vi "メイン.vi"() -> (2 "測定周期/ms":dbl, 3 "値転記用配列":T2[](array[typedef]))   [LabVIEW 2021] (continued)
                      n6047 = property on="MAX/MINグローバルリセット用" class="Arr (指定)"() -> ("Value"=w8245:string[][])  [unwired: 2 in, 2 out]
                      n6048 = global write "測定値MAXMIN_G.vi" "測定値MAX/MINグローバル"(w8245) -> ()
                    }
                  }
                  n6049 = case shown="FALSE" w8244 {
                    frame False {
                    }
                    frame True {
                      n6050 = property on="MAX/MINグローバルリセット用" class="Arr (指定)"() -> ("Value"=w8246:string[][])  [unwired: 2 in, 2 out]
                      n6051 = global write "測定値MAXMIN_G.vi" "測定値MAX/MINグローバル"(w8246) -> ()
                    }
                  }
                }
                frame 1 {
                  n6052 = local read "測定新値\nリセット用 2"() -> (w8247:bool)
                  n6053 = local read "測定旧値 2"() -> (w8248:bool)
                  n6054 = case shown="FALSE" w8247 {
                    frame False {
                    }
                    frame True {
                      n6055 = property on="MAX/MINグローバルリセット用" class="Arr (指定)"() -> ("Value"=w8249:string[][])  [unwired: 2 in, 2 out]
                      n6056 = global write "測定値MAXMIN_G.vi" "測定値MAX/MINグローバル"(w8249) -> ()
                    }
                  }
                  n6057 = case shown="FALSE" w8248 {
                    frame False {
                    }
                    frame True {
                      n6058 = property on="MAX/MINグローバルリセット用" class="Arr (指定)"() -> ("Value"=w8250:string[][])  [unwired: 2 in, 2 out]
                      n6059 = global write "測定値MAXMIN_G.vi" "測定値MAX/MINグローバル"(w8250) -> ()
                    }
                  }
                }
                frame 2 {
                  n6060 = local read "測定新値\nリセット用 3"() -> (w8251:bool)
                  n6061 = local read "測定旧値 3"() -> (w8252:bool)
                  n6062 = case shown="FALSE" w8251 {
                    frame False {
                    }
                    frame True {
                      n6063 = property on="MAX/MINグローバルリセット用" class="Arr (指定)"() -> ("Value"=w8253:string[][])  [unwired: 2 in, 2 out]
                      n6064 = global write "測定値MAXMIN_G.vi" "測定値MAX/MINグローバル"(w8253) -> ()
                    }
                  }
                  n6065 = case shown="FALSE" w8252 {
                    frame False {
                    }
                    frame True {
                      n6066 = property on="MAX/MINグローバルリセット用" class="Arr (指定)"() -> ("Value"=w8254:string[][])  [unwired: 2 in, 2 out]
                      n6067 = global write "測定値MAXMIN_G.vi" "測定値MAX/MINグローバル"(w8254) -> ()
                    }
                  }
                }
                frame 3 {
                  n6068 = local read "測定新値\nリセット用 4"() -> (w8255:bool)
                  n6069 = local read "測定旧値 4"() -> (w8256:bool)
                  n6070 = case shown="FALSE" w8255 {
                    frame False {
                    }
                    frame True {
                      n6071 = property on="MAX/MINグローバルリセット用" class="Arr (指定)"() -> ("Value"=w8257:string[][])  [unwired: 2 in, 2 out]
                      n6072 = global write "測定値MAXMIN_G.vi" "測定値MAX/MINグローバル"(w8257) -> ()
                    }
                  }
                  n6073 = case shown="FALSE" w8256 {
                    frame False {
                    }
                    frame True {
                      n6074 = property on="MAX/MINグローバルリセット用" class="Arr (指定)"() -> ("Value"=w8258:string[][])  [unwired: 2 in, 2 out]
                      n6075 = global write "測定値MAXMIN_G.vi" "測定値MAX/MINグローバル"(w8258) -> ()
                    }
                  }
                }
                frame 4 {
                  n6076 = local read "測定新値\nリセット用 5"() -> (w8259:bool)
                  n6077 = local read "測定旧値 5"() -> (w8260:bool)
                  n6078 = case shown="FALSE" w8259 {
                    frame False {
                    }
                    frame True {
                      n6079 = property on="MAX/MINグローバルリセット用" class="Arr (指定)"() -> ("Value"=w8261:string[][])  [unwired: 2 in, 2 out]
                      n6080 = global write "測定値MAXMIN_G.vi" "測定値MAX/MINグローバル"(w8261) -> ()
                    }
                  }
                  n6081 = case shown="FALSE" w8260 {
                    frame False {
                    }
                    frame True {
                      n6082 = property on="MAX/MINグローバルリセット用" class="Arr (指定)"() -> ("Value"=w8262:string[][])  [unwired: 2 in, 2 out]
                      n6083 = global write "測定値MAXMIN_G.vi" "測定値MAX/MINグローバル"(w8262) -> ()
                    }
                  }
                }
                frame 5 {
                  n6084 = local read "測定新値\nリセット用 6"() -> (w8263:bool)
                  n6085 = local read "測定旧値 6"() -> (w8264:bool)
                  n6086 = case shown="FALSE" w8263 {
                    frame False {
                    }
                    frame True {
                      n6087 = property on="MAX/MINグローバルリセット用" class="Arr (指定)"() -> ("Value"=w8265:string[][])  [unwired: 2 in, 2 out]
                      n6088 = global write "測定値MAXMIN_G.vi" "測定値MAX/MINグローバル"(w8265) -> ()
                    }
                  }
                  n6089 = case shown="FALSE" w8264 {
                    frame False {
                    }
                    frame True {
                      n6090 = property on="MAX/MINグローバルリセット用" class="Arr (指定)"() -> ("Value"=w8266:string[][])  [unwired: 2 in, 2 out]
                      n6091 = global write "測定値MAXMIN_G.vi" "測定値MAX/MINグローバル"(w8266) -> ()
                    }
                  }
                }
                frame 6 {
                  n6092 = local read "測定新値\nリセット用 7"() -> (w8267:bool)
                  n6093 = local read "測定旧値 7"() -> (w8268:bool)
                  n6094 = case shown="FALSE" w8267 {
                    frame False {
                    }
                    frame True {
                      n6095 = property on="MAX/MINグローバルリセット用" class="Arr (指定)"() -> ("Value"=w8269:string[][])  [unwired: 2 in, 2 out]
                      n6096 = global write "測定値MAXMIN_G.vi" "測定値MAX/MINグローバル"(w8269) -> ()
                    }
                  }
                  n6097 = case shown="FALSE" w8268 {
                    frame False {
                    }
                    frame True {
                      n6098 = property on="MAX/MINグローバルリセット用" class="Arr (指定)"() -> ("Value"=w8270:string[][])  [unwired: 2 in, 2 out]
                      n6099 = global write "測定値MAXMIN_G.vi" "測定値MAX/MINグローバル"(w8270) -> ()
                    }
                  }
                }
                frame 7 {
                  n6100 = local read "測定新値\nリセット用 8"() -> (w8271:bool)
                  n6101 = local read "測定旧値 8"() -> (w8272:bool)
                  n6102 = case shown="FALSE" w8271 {
                    frame False {
                    }
                    frame True {
                      n6103 = property on="MAX/MINグローバルリセット用" class="Arr (指定)"() -> ("Value"=w8273:string[][])  [unwired: 2 in, 2 out]
                      n6104 = global write "測定値MAXMIN_G.vi" "測定値MAX/MINグローバル"(w8273) -> ()
                    }
                  }
                  n6105 = case shown="FALSE" w8272 {
                    frame False {
                    }
                    frame True {
                      n6106 = property on="MAX/MINグローバルリセット用" class="Arr (指定)"() -> ("Value"=w8274:string[][])  [unwired: 2 in, 2 out]
                      n6107 = global write "測定値MAXMIN_G.vi" "測定値MAX/MINグローバル"(w8274) -> ()
                    }
                  }
                }
                frame 8 {
                  n6108 = local read "測定新値\nリセット用 9"() -> (w8275:bool)
                  n6109 = local read "測定旧値 9"() -> (w8276:bool)
                  n6110 = case shown="FALSE" w8275 {
                    frame False {
                    }
                    frame True {
                      n6111 = property on="MAX/MINグローバルリセット用" class="Arr (指定)"() -> ("Value"=w8277:string[][])  [unwired: 2 in, 2 out]
                      n6112 = global write "測定値MAXMIN_G.vi" "測定値MAX/MINグローバル"(w8277) -> ()
                    }
                  }
                  n6113 = case shown="FALSE" w8276 {
                    frame False {
                    }
                    frame True {
                      n6114 = property on="MAX/MINグローバルリセット用" class="Arr (指定)"() -> ("Value"=w8278:string[][])  [unwired: 2 in, 2 out]
                      n6115 = global write "測定値MAXMIN_G.vi" "測定値MAX/MINグローバル"(w8278) -> ()
                    }
                  }
                }
                frame 10 {
                  n6116 = local read "測定新値\nリセット用 11"() -> (w8279:bool)
                  n6117 = local read "測定旧値 11"() -> (w8280:bool)
                  n6118 = case shown="FALSE" w8279 {
                    frame False {
                    }
                    frame True {
                      n6119 = property on="MAX/MINグローバルリセット用" class="Arr (指定)"() -> ("Value"=w8281:string[][])  [unwired: 2 in, 2 out]
                      n6120 = global write "測定値MAXMIN_G.vi" "測定値MAX/MINグローバル"(w8281) -> ()
                    }
                  }
                  n6121 = case shown="FALSE" w8280 {
                    frame False {
                    }
                    frame True {
                      n6122 = property on="MAX/MINグローバルリセット用" class="Arr (指定)"() -> ("Value"=w8282:string[][])  [unwired: 2 in, 2 out]
                      n6123 = global write "測定値MAXMIN_G.vi" "測定値MAX/MINグローバル"(w8282) -> ()
                    }
                  }
                }
                frame 11 {
                  n6124 = local read "測定新値\nリセット用 12"() -> (w8283:bool)
                  n6125 = local read "測定旧値 12"() -> (w8284:bool)
                  n6126 = case shown="FALSE" w8283 {
                    frame False {
                    }
                    frame True {
                      n6127 = property on="MAX/MINグローバルリセット用" class="Arr (指定)"() -> ("Value"=w8285:string[][])  [unwired: 2 in, 2 out]
                      n6128 = global write "測定値MAXMIN_G.vi" "測定値MAX/MINグローバル"(w8285) -> ()
                    }
                  }
                  n6129 = case shown="FALSE" w8284 {
                    frame False {
                    }
                    frame True {
                      n6130 = property on="MAX/MINグローバルリセット用" class="Arr (指定)"() -> ("Value"=w8286:string[][])  [unwired: 2 in, 2 out]
                      n6131 = global write "測定値MAXMIN_G.vi" "測定値MAX/MINグローバル"(w8286) -> ()
                    }
                  }
                }
              }
            }
          }
          frame #1 {
            w8287 = FALSE
            # "②測定新規リセット用、測定旧値のリセット"
            n6132 = for {
              N: w8288 -> [_]
              tunnel: w8287 -> [w8292]
              i -> [w8293]
              n6133 = case shown="11" w8293 {
                tunnel: w8292 -> [w8294 w8295 w8296 w8297 w8298 w8299 w8300 w8301 w8302 w8303 w8304 w8305]
                frame 0, Default {
                  n6134 = local write "測定新値\nリセット用 1"(w8294) -> ()
                  n6135 = local write "測定旧値 1"(w8294) -> ()
                }
                frame 1 {
                  n6136 = local write "測定新値\nリセット用 2"(w8295) -> ()
                  n6137 = local write "測定旧値 2"(w8295) -> ()
                }
                frame 2 {
                  n6138 = local write "測定新値\nリセット用 3"(w8296) -> ()
                  n6139 = local write "測定旧値 3"(w8296) -> ()
                }
                frame 3 {
                  n6140 = local write "測定新値\nリセット用 4"(w8297) -> ()
                  n6141 = local write "測定旧値 4"(w8297) -> ()
                }
                frame 4 {
                  n6142 = local write "測定新値\nリセット用 5"(w8298) -> ()
                  n6143 = local write "測定旧値 5"(w8298) -> ()
                }
                frame 5 {
                  n6144 = local write "測定新値\nリセット用 6"(w8299) -> ()
                  n6145 = local write "測定旧値 6"(w8299) -> ()
                }
                frame 6 {
                  n6146 = local write "測定新値\nリセット用 7"(w8300) -> ()
                  n6147 = local write "測定旧値 7"(w8300) -> ()
                }
                frame 7 {
                  n6148 = local write "測定新値\nリセット用 8"(w8301) -> ()
                  n6149 = local write "測定旧値 8"(w8301) -> ()
                }
                frame 8 {
                  n6150 = local write "測定新値\nリセット用 9"(w8302) -> ()
                  n6151 = local write "測定旧値 9"(w8302) -> ()
                }
                frame 9 {
                  n6152 = local write "測定新値\nリセット用 10"(w8303) -> ()
                  n6153 = local write "測定旧値 10"(w8303) -> ()
                }
                frame 10 {
                  n6154 = local write "測定新値\nリセット用 11"(w8304) -> ()
                  n6155 = local write "測定旧値 11"(w8304) -> ()
                }
                frame 11 {
                  n6156 = local write "測定新値\nリセット用 12"(w8305) -> ()
                  n6157 = local write "測定旧値 12"(w8305) -> ()
                }
              }
            }
            n6158 = global write "測定キャンセルボタン.vi" "グローバル_測定キャンセルボタン"(w8287) -> ()
            n6159 = local write "G_メイン測定キャンセルボタン"(w8287) -> ()
          }
          frame #2 {
            # "⑦キュー"
            # "④グローバル_測定キャンセルボタンを\n対象測定新値がFalseならTrueにする"
            n6160 = case shown="TRUE" w8308 {
              tunnel: [_ w8318] -> w8312
              tunnel: w8311 -> [_ w8317]
              tunnel: [_ w8316] -> w8310
              tunnel: w8309 -> [_ w8315]
              tunnel: [w8313 w8314] -> w8307
              tunnel: [w8313 w8314] -> w8306
              frame False {
                w8313 = TRUE
              }
              frame True {
                w8314 = TRUE
                n6161 = Enqueue Element(queue=w8317, element="測定10", error in (no error)=w8315) -> (queue out=w8318:refnum<queue>, error out=w8316:errorcluster)  [unwired: 1 in, 1 out]
              }
            }
            n6162 = local write "G_メイン測定キャンセルボタン"(w8307) -> ()
            n6163 = global write "測定キャンセルボタン.vi" "グローバル_測定キャンセルボタン"(w8306) -> ()
          }
        }
        n6164 = for {
          N: 12 -> [_]
          tunnel: w8210 -> [w8224]
          i -> [w8225]
          n6165 = case shown="11" w8225 {
            tunnel: w8224 -> [w8226 w8227 w8228 w8229 w8230 w8231 w8232 w8233 w8234 w8235 w8236 w8237]
            frame 0, Default {
              n6166 = property on="メイン測定ボタン_単発 1" class="Bool (指定)"("DisabledEnum"=w8226) -> ()  [unwired: 2 in, 2 out]
              n6167 = property on="メイン測定ボタン_連続 1" class="Bool (指定)"("DisabledEnum"=w8226) -> ()  [unwired: 2 in, 2 out]
            }
            frame 1 {
              n6168 = property on="メイン測定ボタン_単発 2" class="Bool (指定)"("DisabledEnum"=w8227) -> ()  [unwired: 2 in, 2 out]
              n6169 = property on="メイン測定ボタン_連続 2" class="Bool (指定)"("DisabledEnum"=w8227) -> ()  [unwired: 2 in, 2 out]
            }
            frame 2 {
              n6170 = property on="メイン測定ボタン_単発 3" class="Bool (指定)"("DisabledEnum"=w8228) -> ()  [unwired: 2 in, 2 out]
              n6171 = property on="メイン測定ボタン_連続 3" class="Bool (指定)"("DisabledEnum"=w8228) -> ()  [unwired: 2 in, 2 out]
            }
            frame 3 {
              n6172 = property on="メイン測定ボタン_単発 4" class="Bool (指定)"("DisabledEnum"=w8229) -> ()  [unwired: 2 in, 2 out]
              n6173 = property on="メイン測定ボタン_連続 4" class="Bool (指定)"("DisabledEnum"=w8229) -> ()  [unwired: 2 in, 2 out]
            }
            frame 4 {
              n6174 = property on="メイン測定ボタン_単発 5" class="Bool (指定)"("DisabledEnum"=w8230) -> ()  [unwired: 2 in, 2 out]
              n6175 = property on="メイン測定ボタン_連続 5" class="Bool (指定)"("DisabledEnum"=w8230) -> ()  [unwired: 2 in, 2 out]
            }
            frame 5 {
              n6176 = property on="メイン測定ボタン_連続 6" class="Bool (指定)"("DisabledEnum"=w8231) -> ()  [unwired: 2 in, 2 out]
              n6177 = property on="メイン測定ボタン_単発 6" class="Bool (指定)"("DisabledEnum"=w8231) -> ()  [unwired: 2 in, 2 out]
            }
            frame 6 {
              n6178 = property on="メイン測定ボタン_連続 7" class="Bool (指定)"("DisabledEnum"=w8232) -> ()  [unwired: 2 in, 2 out]
              n6179 = property on="メイン測定ボタン_単発 7" class="Bool (指定)"("DisabledEnum"=w8232) -> ()  [unwired: 2 in, 2 out]
            }
            frame 7 {
              n6180 = property on="メイン測定ボタン_単発 8" class="Bool (指定)"("DisabledEnum"=w8233) -> ()  [unwired: 2 in, 2 out]
              n6181 = property on="メイン測定ボタン_連続 8" class="Bool (指定)"("DisabledEnum"=w8233) -> ()  [unwired: 2 in, 2 out]
            }
            frame 8 {
              n6182 = property on="メイン測定ボタン_単発 9" class="Bool (指定)"("DisabledEnum"=w8234) -> ()  [unwired: 2 in, 2 out]
              n6183 = property on="メイン測定ボタン_連続 9" class="Bool (指定)"("DisabledEnum"=w8234) -> ()  [unwired: 2 in, 2 out]
            }
            frame 9 {
              n6184 = property on="メイン測定ボタン_単発 10" class="Bool (指定)"("DisabledEnum"=w8235) -> ()  [unwired: 2 in, 2 out]
              n6185 = property on="メイン測定ボタン_連続 10" class="Bool (指定)"("DisabledEnum"=w8235) -> ()  [unwired: 2 in, 2 out]
            }
            frame 10 {
              n6186 = property on="メイン測定ボタン_単発 11" class="Bool (指定)"("DisabledEnum"=w8236) -> ()  [unwired: 2 in, 2 out]
              n6187 = property on="メイン測定ボタン_連続 11" class="Bool (指定)"("DisabledEnum"=w8236) -> ()  [unwired: 2 in, 2 out]
            }
            frame 11 {
              n6188 = property on="メイン測定ボタン_連続 12" class="Bool (指定)"("DisabledEnum"=w8237) -> ()  [unwired: 2 in, 2 out]
              n6189 = property on="メイン測定ボタン_単発 12" class="Bool (指定)"("DisabledEnum"=w8237) -> ()  [unwired: 2 in, 2 out]
            }
          }
        }
        n6190 = property on="TOPページへ" class="Bool"("DisabledEnum"=w8210) -> ()  [unwired: 2 in, 2 out]
        n6191 = property on="保存して終了" class="Bool"("DisabledEnum"=w8210) -> ()  [unwired: 2 in, 2 out]
        n6192 = property on="保存せずに" class="Bool"("DisabledEnum"=w8210) -> ()  [unwired: 2 in, 2 out]
      }
      event Value Change {
        w8322 = T8."Disabled" ("無効")
        # "⑤"
        # "※複製時\n①このボタンで操作する以外の\n測定旧値\n測定新値\nを複製して作る\n②ある分だけの\n測定旧値\nを複製して作る\n③ある分だけの\n測定旧値\nを複製して作る\n④はそのまま\n⑤測定新値の\nボタンが複製されているか確認\n⑥Ⅰ.初期設定の\n測定新値_リセットの初期化\nを必ず作る事\n⑦キュー\n⑧ループカウント"
        # "単発測定ボタンを押した時、G_メインとグローバルのキャンセルボタンがFalseになり、連続測定が可能な状態になる。\n500ミリ秒後G_メインとグローバルのキャンセルボタンがTrueになり、連続測定が止まる"
        n6193 = event-data() -> ("NewVal"=w8321:T7)  [unwired: 1 in, 2 out]
        "測定新値 11" <- w8321
        n6194 = local read "書込周期/ms"() -> (w8320:dbl)
        n6195 = Wait (ms)(milliseconds to wait=w8320) -> ()  [unwired: 1 out]
        n6196 = flat-sequence {
          tunnel: w8321 -> [w8350]
          tunnel: w8331 -> [w8351]
          tunnel: w8333 -> [w8352]
          tunnel: [w8352] -> w8327
          tunnel: [w8351] -> w8326
          tunnel: [w8350] -> w8325
          tunnel: [w8349] -> w8324
          tunnel: [w8402] -> w8330
          tunnel: [w8401] -> w8329
          tunnel: [w8400] -> w8328
          tunnel: w8324 -> [w8399]
          tunnel: w8325 -> [w8400]
          tunnel: w8326 -> [w8401]
          tunnel: w8327 -> [w8402]
          tunnel: [w8423] -> w8334
          tunnel: [w8421] -> w8332
          tunnel: w8330 -> [w8422]
          tunnel: w8329 -> [w8420]
          tunnel: w8328 -> [w8419]
          frame #0 {
            w8349 = 32
            # "測定旧値・新値～32までTrueだったらMAX/MINグローバルリセット"
            # "①"
            n6197 = for {
              N: w8349 -> [_]
              i -> [w8353]
              n6198 = case shown="11" w8353 {
                frame 0, Default {
                  n6199 = local read "測定新値\nリセット用 1"() -> (w8354:bool)
                  n6200 = local read "測定旧値 1"() -> (w8355:bool)
                  n6201 = case shown="FALSE" w8354 {
                    frame False {
                    }
                    frame True {
                      n6202 = property on="MAX/MINグローバルリセット用" class="Arr (指定)"() -> ("Value"=w8356:string[][])  [unwired: 2 in, 2 out]
                      n6203 = global write "測定値MAXMIN_G.vi" "測定値MAX/MINグローバル"(w8356) -> ()
                    }
                  }
                  n6204 = case shown="FALSE" w8355 {
                    frame False {
                    }
                    frame True {
                      n6205 = property on="MAX/MINグローバルリセット用" class="Arr (指定)"() -> ("Value"=w8357:string[][])  [unwired: 2 in, 2 out]
                      n6206 = global write "測定値MAXMIN_G.vi" "測定値MAX/MINグローバル"(w8357) -> ()
                    }
                  }
                }
                frame 1 {
                  n6207 = local read "測定新値\nリセット用 2"() -> (w8358:bool)
                  n6208 = local read "測定旧値 2"() -> (w8359:bool)
                  n6209 = case shown="FALSE" w8358 {
                    frame False {
                    }
                    frame True {
                      n6210 = property on="MAX/MINグローバルリセット用" class="Arr (指定)"() -> ("Value"=w8360:string[][])  [unwired: 2 in, 2 out]
                      n6211 = global write "測定値MAXMIN_G.vi" "測定値MAX/MINグローバル"(w8360) -> ()
                    }
                  }
                  n6212 = case shown="FALSE" w8359 {
                    frame False {
                    }
                    frame True {
                      n6213 = property on="MAX/MINグローバルリセット用" class="Arr (指定)"() -> ("Value"=w8361:string[][])  [unwired: 2 in, 2 out]
                      n6214 = global write "測定値MAXMIN_G.vi" "測定値MAX/MINグローバル"(w8361) -> ()
                    }
                  }
                }
                frame 2 {
                  n6215 = local read "測定新値\nリセット用 3"() -> (w8362:bool)
                  n6216 = local read "測定旧値 3"() -> (w8363:bool)
                  n6217 = case shown="FALSE" w8362 {
                    frame False {
                    }
                    frame True {
                      n6218 = property on="MAX/MINグローバルリセット用" class="Arr (指定)"() -> ("Value"=w8364:string[][])  [unwired: 2 in, 2 out]
                      n6219 = global write "測定値MAXMIN_G.vi" "測定値MAX/MINグローバル"(w8364) -> ()
                    }
                  }
                  n6220 = case shown="FALSE" w8363 {
                    frame False {
                    }
                    frame True {
                      n6221 = property on="MAX/MINグローバルリセット用" class="Arr (指定)"() -> ("Value"=w8365:string[][])  [unwired: 2 in, 2 out]
                      n6222 = global write "測定値MAXMIN_G.vi" "測定値MAX/MINグローバル"(w8365) -> ()
                    }
                  }
                }
                frame 3 {
                  n6223 = local read "測定新値\nリセット用 4"() -> (w8366:bool)
                  n6224 = local read "測定旧値 4"() -> (w8367:bool)
                  n6225 = case shown="FALSE" w8366 {
                    frame False {
                    }
                    frame True {
                      n6226 = property on="MAX/MINグローバルリセット用" class="Arr (指定)"() -> ("Value"=w8368:string[][])  [unwired: 2 in, 2 out]
                      n6227 = global write "測定値MAXMIN_G.vi" "測定値MAX/MINグローバル"(w8368) -> ()
                    }
                  }
                  n6228 = case shown="FALSE" w8367 {
                    frame False {
                    }
                    frame True {
                      n6229 = property on="MAX/MINグローバルリセット用" class="Arr (指定)"() -> ("Value"=w8369:string[][])  [unwired: 2 in, 2 out]
                      n6230 = global write "測定値MAXMIN_G.vi" "測定値MAX/MINグローバル"(w8369) -> ()
                    }
                  }
                }
                frame 4 {
                  n6231 = local read "測定新値\nリセット用 5"() -> (w8370:bool)
                  n6232 = local read "測定旧値 5"() -> (w8371:bool)
                  n6233 = case shown="FALSE" w8370 {
                    frame False {
                    }
                    frame True {
                      n6234 = property on="MAX/MINグローバルリセット用" class="Arr (指定)"() -> ("Value"=w8372:string[][])  [unwired: 2 in, 2 out]
                      n6235 = global write "測定値MAXMIN_G.vi" "測定値MAX/MINグローバル"(w8372) -> ()
                    }
                  }
                  n6236 = case shown="FALSE" w8371 {
                    frame False {
                    }
                    frame True {
                      n6237 = property on="MAX/MINグローバルリセット用" class="Arr (指定)"() -> ("Value"=w8373:string[][])  [unwired: 2 in, 2 out]
                      n6238 = global write "測定値MAXMIN_G.vi" "測定値MAX/MINグローバル"(w8373) -> ()
                    }
                  }
                }
                frame 5 {
                  n6239 = local read "測定新値\nリセット用 6"() -> (w8374:bool)
                  n6240 = local read "測定旧値 6"() -> (w8375:bool)
                  n6241 = case shown="FALSE" w8374 {
                    frame False {
                    }
                    frame True {
                      n6242 = property on="MAX/MINグローバルリセット用" class="Arr (指定)"() -> ("Value"=w8376:string[][])  [unwired: 2 in, 2 out]
                      n6243 = global write "測定値MAXMIN_G.vi" "測定値MAX/MINグローバル"(w8376) -> ()
                    }
                  }
                  n6244 = case shown="FALSE" w8375 {
                    frame False {
                    }
                    frame True {
                      n6245 = property on="MAX/MINグローバルリセット用" class="Arr (指定)"() -> ("Value"=w8377:string[][])  [unwired: 2 in, 2 out]
                      n6246 = global write "測定値MAXMIN_G.vi" "測定値MAX/MINグローバル"(w8377) -> ()
                    }
                  }
                }
                frame 6 {
                  n6247 = local read "測定新値\nリセット用 7"() -> (w8378:bool)
                  n6248 = local read "測定旧値 7"() -> (w8379:bool)
                  n6249 = case shown="FALSE" w8378 {
                    frame False {
                    }
                    frame True {
                      n6250 = property on="MAX/MINグローバルリセット用" class="Arr (指定)"() -> ("Value"=w8380:string[][])  [unwired: 2 in, 2 out]
                      n6251 = global write "測定値MAXMIN_G.vi" "測定値MAX/MINグローバル"(w8380) -> ()
                    }
                  }
                  n6252 = case shown="FALSE" w8379 {
                    frame False {
                    }
                    frame True {
                      n6253 = property on="MAX/MINグローバルリセット用" class="Arr (指定)"() -> ("Value"=w8381:string[][])  [unwired: 2 in, 2 out]
                      n6254 = global write "測定値MAXMIN_G.vi" "測定値MAX/MINグローバル"(w8381) -> ()
                    }
                  }
                }
                frame 7 {
                  n6255 = local read "測定新値\nリセット用 8"() -> (w8382:bool)
                  n6256 = local read "測定旧値 8"() -> (w8383:bool)
                  n6257 = case shown="FALSE" w8382 {
                    frame False {
                    }
                    frame True {
                      n6258 = property on="MAX/MINグローバルリセット用" class="Arr (指定)"() -> ("Value"=w8384:string[][])  [unwired: 2 in, 2 out]
                      n6259 = global write "測定値MAXMIN_G.vi" "測定値MAX/MINグローバル"(w8384) -> ()
                    }
                  }
                  n6260 = case shown="FALSE" w8383 {
                    frame False {
                    }
                    frame True {
                      n6261 = property on="MAX/MINグローバルリセット用" class="Arr (指定)"() -> ("Value"=w8385:string[][])  [unwired: 2 in, 2 out]
                      n6262 = global write "測定値MAXMIN_G.vi" "測定値MAX/MINグローバル"(w8385) -> ()
                    }
                  }
                }
                frame 8 {
                  n6263 = local read "測定新値\nリセット用 9"() -> (w8386:bool)
                  n6264 = local read "測定旧値 9"() -> (w8387:bool)
                  n6265 = case shown="FALSE" w8386 {
                    frame False {
                    }
                    frame True {
                      n6266 = property on="MAX/MINグローバルリセット用" class="Arr (指定)"() -> ("Value"=w8388:string[][])  [unwired: 2 in, 2 out]
                      n6267 = global write "測定値MAXMIN_G.vi" "測定値MAX/MINグローバル"(w8388) -> ()
                    }
                  }
                  n6268 = case shown="FALSE" w8387 {
                    frame False {
                    }
                    frame True {
                      n6269 = property on="MAX/MINグローバルリセット用" class="Arr (指定)"() -> ("Value"=w8389:string[][])  [unwired: 2 in, 2 out]
                      n6270 = global write "測定値MAXMIN_G.vi" "測定値MAX/MINグローバル"(w8389) -> ()
                    }
                  }
                }
                frame 9 {
                  n6271 = local read "測定新値\nリセット用 10"() -> (w8390:bool)
                  n6272 = local read "測定旧値 10"() -> (w8391:bool)
                  n6273 = case shown="FALSE" w8390 {
                    frame False {
                    }
                    frame True {
                      n6274 = property on="MAX/MINグローバルリセット用" class="Arr (指定)"() -> ("Value"=w8392:string[][])  [unwired: 2 in, 2 out]
                      n6275 = global write "測定値MAXMIN_G.vi" "測定値MAX/MINグローバル"(w8392) -> ()
                    }
                  }
                  n6276 = case shown="FALSE" w8391 {
                    frame False {
                    }
                    frame True {
                      n6277 = property on="MAX/MINグローバルリセット用" class="Arr (指定)"() -> ("Value"=w8393:string[][])  [unwired: 2 in, 2 out]
                      n6278 = global write "測定値MAXMIN_G.vi" "測定値MAX/MINグローバル"(w8393) -> ()
                    }
                  }
                }
                frame 11 {
                  n6279 = local read "測定新値\nリセット用 12"() -> (w8394:bool)
                  n6280 = local read "測定旧値 12"() -> (w8395:bool)
                  n6281 = case shown="FALSE" w8394 {
                    frame False {
                    }
                    frame True {
                      n6282 = property on="MAX/MINグローバルリセット用" class="Arr (指定)"() -> ("Value"=w8396:string[][])  [unwired: 2 in, 2 out]
                      n6283 = global write "測定値MAXMIN_G.vi" "測定値MAX/MINグローバル"(w8396) -> ()
                    }
                  }
                  n6284 = case shown="FALSE" w8395 {
                    frame False {
                    }
                    frame True {
                      n6285 = property on="MAX/MINグローバルリセット用" class="Arr (指定)"() -> ("Value"=w8397:string[][])  [unwired: 2 in, 2 out]
                      n6286 = global write "測定値MAXMIN_G.vi" "測定値MAX/MINグローバル"(w8397) -> ()
                    }
                  }
                }
              }
            }
          }
          frame #1 {
            w8398 = FALSE
            # "②測定新規リセット用、測定旧値のリセット"
            n6287 = for {
              N: w8399 -> [_]
              tunnel: w8398 -> [w8403]
              i -> [w8404]
              n6288 = case shown="11" w8404 {
                tunnel: w8403 -> [w8405 w8406 w8407 w8408 w8409 w8410 w8411 w8412 w8413 w8414 w8415 w8416]
                frame 0, Default {
                  n6289 = local write "測定新値\nリセット用 1"(w8405) -> ()
                  n6290 = local write "測定旧値 1"(w8405) -> ()
                }
                frame 1 {
                  n6291 = local write "測定新値\nリセット用 2"(w8406) -> ()
                  n6292 = local write "測定旧値 2"(w8406) -> ()
                }
                frame 2 {
                  n6293 = local write "測定新値\nリセット用 3"(w8407) -> ()
                  n6294 = local write "測定旧値 3"(w8407) -> ()
                }
                frame 3 {
                  n6295 = local write "測定新値\nリセット用 4"(w8408) -> ()
                  n6296 = local write "測定旧値 4"(w8408) -> ()
                }
                frame 4 {
                  n6297 = local write "測定新値\nリセット用 5"(w8409) -> ()
                  n6298 = local write "測定旧値 5"(w8409) -> ()
                }
                frame 5 {
                  n6299 = local write "測定新値\nリセット用 6"(w8410) -> ()
                  n6300 = local write "測定旧値 6"(w8410) -> ()
                }
                frame 6 {
                  n6301 = local write "測定新値\nリセット用 7"(w8411) -> ()
                  n6302 = local write "測定旧値 7"(w8411) -> ()
                }
                frame 7 {
                  n6303 = local write "測定新値\nリセット用 8"(w8412) -> ()
                  n6304 = local write "測定旧値 8"(w8412) -> ()
                }
                frame 8 {
                  n6305 = local write "測定新値\nリセット用 9"(w8413) -> ()
                  n6306 = local write "測定旧値 9"(w8413) -> ()
                }
                frame 9 {
                  n6307 = local write "測定新値\nリセット用 10"(w8414) -> ()
                  n6308 = local write "測定旧値 10"(w8414) -> ()
                }
                frame 10 {
                  n6309 = local write "測定新値\nリセット用 11"(w8415) -> ()
                  n6310 = local write "測定旧値 11"(w8415) -> ()
                }
                frame 11 {
                  n6311 = local write "測定新値\nリセット用 12"(w8416) -> ()
                  n6312 = local write "測定旧値 12"(w8416) -> ()
                }
              }
            }
            n6313 = global write "測定キャンセルボタン.vi" "グローバル_測定キャンセルボタン"(w8398) -> ()
            n6314 = local write "G_メイン測定キャンセルボタン"(w8398) -> ()
          }
          frame #2 {
            # "⑦キュー"
            # "④グローバル_測定キャンセルボタンを\n対象測定新値がFalseならTrueにする"
            n6315 = case shown="TRUE" w8419 {
              tunnel: [_ w8429] -> w8423
              tunnel: w8422 -> [_ w8428]
              tunnel: [_ w8427] -> w8421
              tunnel: w8420 -> [_ w8426]
              tunnel: [w8424 w8425] -> w8418
              tunnel: [w8424 w8425] -> w8417
              frame False {
                w8424 = TRUE
              }
              frame True {
                w8425 = TRUE
                n6316 = Enqueue Element(queue=w8428, element="測定11", error in (no error)=w8426) -> (queue out=w8429:refnum<queue>, error out=w8427:errorcluster)  [unwired: 1 in, 1 out]
              }
            }
            n6317 = local write "G_メイン測定キャンセルボタン"(w8418) -> ()
            n6318 = global write "測定キャンセルボタン.vi" "グローバル_測定キャンセルボタン"(w8417) -> ()
          }
        }
        n6319 = for {
          N: 12 -> [_]
          tunnel: w8322 -> [w8335]
          i -> [w8336]
          n6320 = case shown="11" w8336 {
            tunnel: w8335 -> [w8337 w8338 w8339 w8340 w8341 w8342 w8343 w8344 w8345 w8346 w8347 w8348]
            frame 0, Default {
              n6321 = property on="メイン測定ボタン_単発 1" class="Bool (指定)"("DisabledEnum"=w8337) -> ()  [unwired: 2 in, 2 out]
              n6322 = property on="メイン測定ボタン_連続 1" class="Bool (指定)"("DisabledEnum"=w8337) -> ()  [unwired: 2 in, 2 out]
            }
            frame 1 {
              n6323 = property on="メイン測定ボタン_単発 2" class="Bool (指定)"("DisabledEnum"=w8338) -> ()  [unwired: 2 in, 2 out]
              n6324 = property on="メイン測定ボタン_連続 2" class="Bool (指定)"("DisabledEnum"=w8338) -> ()  [unwired: 2 in, 2 out]
            }
            frame 2 {
              n6325 = property on="メイン測定ボタン_単発 3" class="Bool (指定)"("DisabledEnum"=w8339) -> ()  [unwired: 2 in, 2 out]
              n6326 = property on="メイン測定ボタン_連続 3" class="Bool (指定)"("DisabledEnum"=w8339) -> ()  [unwired: 2 in, 2 out]
            }
            frame 3 {
              n6327 = property on="メイン測定ボタン_単発 4" class="Bool (指定)"("DisabledEnum"=w8340) -> ()  [unwired: 2 in, 2 out]
              n6328 = property on="メイン測定ボタン_連続 4" class="Bool (指定)"("DisabledEnum"=w8340) -> ()  [unwired: 2 in, 2 out]
            }
            frame 4 {
              n6329 = property on="メイン測定ボタン_単発 5" class="Bool (指定)"("DisabledEnum"=w8341) -> ()  [unwired: 2 in, 2 out]
              n6330 = property on="メイン測定ボタン_連続 5" class="Bool (指定)"("DisabledEnum"=w8341) -> ()  [unwired: 2 in, 2 out]
            }
            frame 5 {
              n6331 = property on="メイン測定ボタン_連続 6" class="Bool (指定)"("DisabledEnum"=w8342) -> ()  [unwired: 2 in, 2 out]
              n6332 = property on="メイン測定ボタン_単発 6" class="Bool (指定)"("DisabledEnum"=w8342) -> ()  [unwired: 2 in, 2 out]
            }
            frame 6 {
              n6333 = property on="メイン測定ボタン_連続 7" class="Bool (指定)"("DisabledEnum"=w8343) -> ()  [unwired: 2 in, 2 out]
              n6334 = property on="メイン測定ボタン_単発 7" class="Bool (指定)"("DisabledEnum"=w8343) -> ()  [unwired: 2 in, 2 out]
            }
            frame 7 {
              n6335 = property on="メイン測定ボタン_単発 8" class="Bool (指定)"("DisabledEnum"=w8344) -> ()  [unwired: 2 in, 2 out]
              n6336 = property on="メイン測定ボタン_連続 8" class="Bool (指定)"("DisabledEnum"=w8344) -> ()  [unwired: 2 in, 2 out]
            }
            frame 8 {
              n6337 = property on="メイン測定ボタン_単発 9" class="Bool (指定)"("DisabledEnum"=w8345) -> ()  [unwired: 2 in, 2 out]
              n6338 = property on="メイン測定ボタン_連続 9" class="Bool (指定)"("DisabledEnum"=w8345) -> ()  [unwired: 2 in, 2 out]
            }
            frame 9 {
              n6339 = property on="メイン測定ボタン_単発 10" class="Bool (指定)"("DisabledEnum"=w8346) -> ()  [unwired: 2 in, 2 out]
              n6340 = property on="メイン測定ボタン_連続 10" class="Bool (指定)"("DisabledEnum"=w8346) -> ()  [unwired: 2 in, 2 out]
            }
            frame 10 {
              n6341 = property on="メイン測定ボタン_単発 11" class="Bool (指定)"("DisabledEnum"=w8347) -> ()  [unwired: 2 in, 2 out]
              n6342 = property on="メイン測定ボタン_連続 11" class="Bool (指定)"("DisabledEnum"=w8347) -> ()  [unwired: 2 in, 2 out]
            }
            frame 11 {
              n6343 = property on="メイン測定ボタン_連続 12" class="Bool (指定)"("DisabledEnum"=w8348) -> ()  [unwired: 2 in, 2 out]
              n6344 = property on="メイン測定ボタン_単発 12" class="Bool (指定)"("DisabledEnum"=w8348) -> ()  [unwired: 2 in, 2 out]
            }
          }
        }
        n6345 = property on="TOPページへ" class="Bool"("DisabledEnum"=w8322) -> ()  [unwired: 2 in, 2 out]
        n6346 = property on="保存して終了" class="Bool"("DisabledEnum"=w8322) -> ()  [unwired: 2 in, 2 out]
        n6347 = property on="保存せずに" class="Bool"("DisabledEnum"=w8322) -> ()  [unwired: 2 in, 2 out]
      }
      event Value Change {
        w8433 = T8."Disabled" ("無効")
        # "⑤"
        # "※複製時\n①このボタンで操作する以外の\n測定旧値\n測定新値\nを複製して作る\n②ある分だけの\n測定旧値\nを複製して作る\n③ある分だけの\n測定旧値\nを複製して作る\n④はそのまま\n⑤測定新値の\nボタンが複製されているか確認\n⑥Ⅰ.初期設定の\n測定新値_リセットの初期化\nを必ず作る事\n⑦キュー\n⑧ループカウント"
        # "単発測定ボタンを押した時、G_メインとグローバルのキャンセルボタンがFalseになり、連続測定が可能な状態になる。\n500ミリ秒後G_メインとグローバルのキャンセルボタンがTrueになり、連続測定が止まる"
        n6348 = event-data() -> ("NewVal"=w8432:T7)  [unwired: 1 in, 2 out]
        "測定新値 12" <- w8432
        n6349 = local read "書込周期/ms"() -> (w8431:dbl)
        n6350 = Wait (ms)(milliseconds to wait=w8431) -> ()  [unwired: 1 out]
        n6351 = flat-sequence {
          tunnel: w8432 -> [w8461]
          tunnel: w8442 -> [w8462]
          tunnel: w8444 -> [w8463]
          tunnel: [w8463] -> w8438
          tunnel: [w8462] -> w8437
          tunnel: [w8461] -> w8436
          tunnel: [w8460] -> w8435
          tunnel: [w8513] -> w8441
          tunnel: [w8512] -> w8440
          tunnel: [w8511] -> w8439
          tunnel: w8435 -> [w8510]
          tunnel: w8436 -> [w8511]
          tunnel: w8437 -> [w8512]
          tunnel: w8438 -> [w8513]
          tunnel: [w8534] -> w8445
          tunnel: [w8532] -> w8443
          tunnel: w8441 -> [w8533]
          tunnel: w8440 -> [w8531]
          tunnel: w8439 -> [w8530]
          frame #0 {
            w8460 = 32
            # "測定旧値・新値～32までTrueだったらMAX/MINグローバルリセット"
            # "①"
            n6352 = for {
              N: w8460 -> [_]
              i -> [w8464]
              n6353 = case shown="0, デフォルト" w8464 {
                frame 0, Default {
                  n6354 = local read "測定新値\nリセット用 1"() -> (w8465:bool)
                  n6355 = local read "測定旧値 1"() -> (w8466:bool)
                  n6356 = case shown="FALSE" w8465 {
                    frame False {
                    }
                    frame True {
                      n6357 = property on="MAX/MINグローバルリセット用" class="Arr (指定)"() -> ("Value"=w8467:string[][])  [unwired: 2 in, 2 out]
                      n6358 = global write "測定値MAXMIN_G.vi" "測定値MAX/MINグローバル"(w8467) -> ()
                    }
                  }
                  n6359 = case shown="TRUE" w8466 {
                    frame False {
                    }
                    frame True {
                      n6360 = property on="MAX/MINグローバルリセット用" class="Arr (指定)"() -> ("Value"=w8468:string[][])  [unwired: 2 in, 2 out]
                      n6361 = global write "測定値MAXMIN_G.vi" "測定値MAX/MINグローバル"(w8468) -> ()
                    }
                  }
                }
                frame 1 {
                  n6362 = local read "測定新値\nリセット用 2"() -> (w8469:bool)
                  n6363 = local read "測定旧値 2"() -> (w8470:bool)
                  n6364 = case shown="FALSE" w8469 {
                    frame False {
                    }
                    frame True {
                      n6365 = property on="MAX/MINグローバルリセット用" class="Arr (指定)"() -> ("Value"=w8471:string[][])  [unwired: 2 in, 2 out]
                      n6366 = global write "測定値MAXMIN_G.vi" "測定値MAX/MINグローバル"(w8471) -> ()
                    }
                  }
                  n6367 = case shown="FALSE" w8470 {
                    frame False {
                    }
                    frame True {
                      n6368 = property on="MAX/MINグローバルリセット用" class="Arr (指定)"() -> ("Value"=w8472:string[][])  [unwired: 2 in, 2 out]
                      n6369 = global write "測定値MAXMIN_G.vi" "測定値MAX/MINグローバル"(w8472) -> ()
                    }
                  }
                }
                frame 2 {
                  n6370 = local read "測定新値\nリセット用 3"() -> (w8473:bool)
                  n6371 = local read "測定旧値 3"() -> (w8474:bool)
                  n6372 = case shown="FALSE" w8473 {
                    frame False {
                    }
                    frame True {
                      n6373 = property on="MAX/MINグローバルリセット用" class="Arr (指定)"() -> ("Value"=w8475:string[][])  [unwired: 2 in, 2 out]
                      n6374 = global write "測定値MAXMIN_G.vi" "測定値MAX/MINグローバル"(w8475) -> ()
                    }
                  }
                  n6375 = case shown="FALSE" w8474 {
                    frame False {
                    }
                    frame True {
                      n6376 = property on="MAX/MINグローバルリセット用" class="Arr (指定)"() -> ("Value"=w8476:string[][])  [unwired: 2 in, 2 out]
                      n6377 = global write "測定値MAXMIN_G.vi" "測定値MAX/MINグローバル"(w8476) -> ()
                    }
                  }
                }
                frame 3 {
                  n6378 = local read "測定新値\nリセット用 4"() -> (w8477:bool)
                  n6379 = local read "測定旧値 4"() -> (w8478:bool)
                  n6380 = case shown="FALSE" w8477 {
                    frame False {
                    }
                    frame True {
                      n6381 = property on="MAX/MINグローバルリセット用" class="Arr (指定)"() -> ("Value"=w8479:string[][])  [unwired: 2 in, 2 out]
                      n6382 = global write "測定値MAXMIN_G.vi" "測定値MAX/MINグローバル"(w8479) -> ()
                    }
                  }
                  n6383 = case shown="FALSE" w8478 {
                    frame False {
                    }
                    frame True {
                      n6384 = property on="MAX/MINグローバルリセット用" class="Arr (指定)"() -> ("Value"=w8480:string[][])  [unwired: 2 in, 2 out]
                      n6385 = global write "測定値MAXMIN_G.vi" "測定値MAX/MINグローバル"(w8480) -> ()
                    }
                  }
                }
                frame 4 {
                  n6386 = local read "測定新値\nリセット用 5"() -> (w8481:bool)
                  n6387 = local read "測定旧値 5"() -> (w8482:bool)
                  n6388 = case shown="FALSE" w8481 {
                    frame False {
                    }
                    frame True {
                      n6389 = property on="MAX/MINグローバルリセット用" class="Arr (指定)"() -> ("Value"=w8483:string[][])  [unwired: 2 in, 2 out]
                      n6390 = global write "測定値MAXMIN_G.vi" "測定値MAX/MINグローバル"(w8483) -> ()
                    }
                  }
                  n6391 = case shown="FALSE" w8482 {
                    frame False {
                    }
                    frame True {
                      n6392 = property on="MAX/MINグローバルリセット用" class="Arr (指定)"() -> ("Value"=w8484:string[][])  [unwired: 2 in, 2 out]
                      n6393 = global write "測定値MAXMIN_G.vi" "測定値MAX/MINグローバル"(w8484) -> ()
                    }
                  }
                }
                frame 5 {
                  n6394 = local read "測定新値\nリセット用 6"() -> (w8485:bool)
                  n6395 = local read "測定旧値 6"() -> (w8486:bool)
                  n6396 = case shown="FALSE" w8485 {
                    frame False {
                    }
                    frame True {
                      n6397 = property on="MAX/MINグローバルリセット用" class="Arr (指定)"() -> ("Value"=w8487:string[][])  [unwired: 2 in, 2 out]
                      n6398 = global write "測定値MAXMIN_G.vi" "測定値MAX/MINグローバル"(w8487) -> ()
                    }
                  }
                  n6399 = case shown="FALSE" w8486 {
                    frame False {
                    }
                    frame True {
                      n6400 = property on="MAX/MINグローバルリセット用" class="Arr (指定)"() -> ("Value"=w8488:string[][])  [unwired: 2 in, 2 out]
                      n6401 = global write "測定値MAXMIN_G.vi" "測定値MAX/MINグローバル"(w8488) -> ()
                    }
                  }
                }
                frame 6 {
                  n6402 = local read "測定新値\nリセット用 7"() -> (w8489:bool)
                  n6403 = local read "測定旧値 7"() -> (w8490:bool)
                  n6404 = case shown="FALSE" w8489 {
                    frame False {
                    }
                    frame True {
                      n6405 = property on="MAX/MINグローバルリセット用" class="Arr (指定)"() -> ("Value"=w8491:string[][])  [unwired: 2 in, 2 out]
                      n6406 = global write "測定値MAXMIN_G.vi" "測定値MAX/MINグローバル"(w8491) -> ()
                    }
                  }
                  n6407 = case shown="FALSE" w8490 {
                    frame False {
                    }
                    frame True {
                      n6408 = property on="MAX/MINグローバルリセット用" class="Arr (指定)"() -> ("Value"=w8492:string[][])  [unwired: 2 in, 2 out]
                      n6409 = global write "測定値MAXMIN_G.vi" "測定値MAX/MINグローバル"(w8492) -> ()
                    }
                  }
                }
                frame 7 {
                  n6410 = local read "測定新値\nリセット用 8"() -> (w8493:bool)
                  n6411 = local read "測定旧値 8"() -> (w8494:bool)
                  n6412 = case shown="FALSE" w8493 {
                    frame False {
                    }
                    frame True {
                      n6413 = property on="MAX/MINグローバルリセット用" class="Arr (指定)"() -> ("Value"=w8495:string[][])  [unwired: 2 in, 2 out]
                      n6414 = global write "測定値MAXMIN_G.vi" "測定値MAX/MINグローバル"(w8495) -> ()
                    }
                  }
                  n6415 = case shown="FALSE" w8494 {
                    frame False {
                    }
                    frame True {
                      n6416 = property on="MAX/MINグローバルリセット用" class="Arr (指定)"() -> ("Value"=w8496:string[][])  [unwired: 2 in, 2 out]
                      n6417 = global write "測定値MAXMIN_G.vi" "測定値MAX/MINグローバル"(w8496) -> ()
                    }
                  }
                }
                frame 8 {
                  n6418 = local read "測定新値\nリセット用 9"() -> (w8497:bool)
                  n6419 = local read "測定旧値 9"() -> (w8498:bool)
                  n6420 = case shown="FALSE" w8497 {
                    frame False {
                    }
                    frame True {
                      n6421 = property on="MAX/MINグローバルリセット用" class="Arr (指定)"() -> ("Value"=w8499:string[][])  [unwired: 2 in, 2 out]
                      n6422 = global write "測定値MAXMIN_G.vi" "測定値MAX/MINグローバル"(w8499) -> ()
                    }
                  }
                  n6423 = case shown="FALSE" w8498 {
                    frame False {
                    }
                    frame True {
                      n6424 = property on="MAX/MINグローバルリセット用" class="Arr (指定)"() -> ("Value"=w8500:string[][])  [unwired: 2 in, 2 out]
                      n6425 = global write "測定値MAXMIN_G.vi" "測定値MAX/MINグローバル"(w8500) -> ()
                    }
                  }
                }
                frame 9 {
                  n6426 = local read "測定新値\nリセット用 10"() -> (w8501:bool)
                  n6427 = local read "測定旧値 10"() -> (w8502:bool)
                  n6428 = case shown="FALSE" w8501 {
                    frame False {
                    }
                    frame True {
                      n6429 = property on="MAX/MINグローバルリセット用" class="Arr (指定)"() -> ("Value"=w8503:string[][])  [unwired: 2 in, 2 out]
                      n6430 = global write "測定値MAXMIN_G.vi" "測定値MAX/MINグローバル"(w8503) -> ()
                    }
                  }
                  n6431 = case shown="FALSE" w8502 {
                    frame False {
                    }
                    frame True {
                      n6432 = property on="MAX/MINグローバルリセット用" class="Arr (指定)"() -> ("Value"=w8504:string[][])  [unwired: 2 in, 2 out]
                      n6433 = global write "測定値MAXMIN_G.vi" "測定値MAX/MINグローバル"(w8504) -> ()
                    }
                  }
                }
                frame 10 {
                  n6434 = local read "測定新値\nリセット用 11"() -> (w8505:bool)
                  n6435 = local read "測定旧値 11"() -> (w8506:bool)
                  n6436 = case shown="TRUE" w8505 {
                    frame False {
                    }
                    frame True {
                      n6437 = property on="MAX/MINグローバルリセット用" class="Arr (指定)"() -> ("Value"=w8507:string[][])  [unwired: 2 in, 2 out]
                      n6438 = global write "測定値MAXMIN_G.vi" "測定値MAX/MINグローバル"(w8507) -> ()
                    }
                  }
                  n6439 = case shown="TRUE" w8506 {
                    frame False {
                    }
                    frame True {
                      n6440 = property on="MAX/MINグローバルリセット用" class="Arr (指定)"() -> ("Value"=w8508:string[][])  [unwired: 2 in, 2 out]
                      n6441 = global write "測定値MAXMIN_G.vi" "測定値MAX/MINグローバル"(w8508) -> ()
                    }
                  }
                }
                frame 11 {
                }
              }
            }
          }
          frame #1 {
            w8509 = FALSE
            # "②測定新規リセット用、測定旧値のリセット"
            n6442 = global write "測定キャンセルボタン.vi" "グローバル_測定キャンセルボタン"(w8509) -> ()
            n6443 = local write "G_メイン測定キャンセルボタン"(w8509) -> ()
            n6444 = for {
              N: w8510 -> [_]
              tunnel: w8509 -> [w8514]
              i -> [w8515]
              n6445 = case shown="0, デフォルト" w8515 {
                tunnel: w8514 -> [w8516 w8517 w8518 w8519 w8520 w8521 w8522 w8523 w8524 w8525 w8526 w8527]
                frame 0, Default {
                  n6446 = local write "測定新値\nリセット用 1"(w8516) -> ()
                  n6447 = local write "測定旧値 1"(w8516) -> ()
                }
                frame 1 {
                  n6448 = local write "測定新値\nリセット用 2"(w8517) -> ()
                  n6449 = local write "測定旧値 2"(w8517) -> ()
                }
                frame 2 {
                  n6450 = local write "測定新値\nリセット用 3"(w8518) -> ()
                  n6451 = local write "測定旧値 3"(w8518) -> ()
                }
                frame 3 {
                  n6452 = local write "測定新値\nリセット用 4"(w8519) -> ()
                  n6453 = local write "測定旧値 4"(w8519) -> ()
                }
                frame 4 {
                  n6454 = local write "測定新値\nリセット用 5"(w8520) -> ()
                  n6455 = local write "測定旧値 5"(w8520) -> ()
                }
                frame 5 {
                  n6456 = local write "測定新値\nリセット用 6"(w8521) -> ()
                  n6457 = local write "測定旧値 6"(w8521) -> ()
                }
                frame 6 {
                  n6458 = local write "測定新値\nリセット用 7"(w8522) -> ()
                  n6459 = local write "測定旧値 7"(w8522) -> ()
                }
                frame 7 {
                  n6460 = local write "測定新値\nリセット用 8"(w8523) -> ()
                  n6461 = local write "測定旧値 8"(w8523) -> ()
                }
                frame 8 {
                  n6462 = local write "測定新値\nリセット用 9"(w8524) -> ()
                  n6463 = local write "測定旧値 9"(w8524) -> ()
                }
                frame 9 {
                  n6464 = local write "測定新値\nリセット用 10"(w8525) -> ()
                  n6465 = local write "測定旧値 10"(w8525) -> ()
                }
                frame 10 {
                  n6466 = local write "測定新値\nリセット用 11"(w8526) -> ()
                  n6467 = local write "測定旧値 11"(w8526) -> ()
                }
                frame 11 {
                  n6468 = local write "測定新値\nリセット用 12"(w8527) -> ()
                  n6469 = local write "測定旧値 12"(w8527) -> ()
                }
              }
            }
          }
          frame #2 {
            # "⑦キュー"
            # "④グローバル_測定キャンセルボタンを\n対象測定新値がFalseならTrueにする"
            n6470 = case shown="TRUE" w8530 {
              tunnel: [_ w8540] -> w8534
              tunnel: w8533 -> [_ w8539]
              tunnel: [_ w8538] -> w8532
              tunnel: w8531 -> [_ w8537]
              tunnel: [w8535 w8536] -> w8529
              tunnel: [w8535 w8536] -> w8528
              frame False {
                w8535 = TRUE
              }
              frame True {
                w8536 = TRUE
                n6471 = Enqueue Element(queue=w8539, element="測定12", error in (no error)=w8537) -> (queue out=w8540:refnum<queue>, error out=w8538:errorcluster)  [unwired: 1 in, 1 out]
              }
            }
            n6472 = local write "G_メイン測定キャンセルボタン"(w8529) -> ()
            n6473 = global write "測定キャンセルボタン.vi" "グローバル_測定キャンセルボタン"(w8528) -> ()
          }
        }
        n6474 = for {
          N: 12 -> [_]
          tunnel: w8433 -> [w8446]
          i -> [w8447]
          n6475 = case shown="0, デフォルト" w8447 {
            tunnel: w8446 -> [w8448 w8449 w8450 w8451 w8452 w8453 w8454 w8455 w8456 w8457 w8458 w8459]
            frame 0, Default {
              n6476 = property on="メイン測定ボタン_単発 1" class="Bool (指定)"("DisabledEnum"=w8448) -> ()  [unwired: 2 in, 2 out]
              n6477 = property on="メイン測定ボタン_連続 1" class="Bool (指定)"("DisabledEnum"=w8448) -> ()  [unwired: 2 in, 2 out]
            }
            frame 1 {
              n6478 = property on="メイン測定ボタン_単発 2" class="Bool (指定)"("DisabledEnum"=w8449) -> ()  [unwired: 2 in, 2 out]
              n6479 = property on="メイン測定ボタン_連続 2" class="Bool (指定)"("DisabledEnum"=w8449) -> ()  [unwired: 2 in, 2 out]
            }
            frame 2 {
              n6480 = property on="メイン測定ボタン_単発 3" class="Bool (指定)"("DisabledEnum"=w8450) -> ()  [unwired: 2 in, 2 out]
              n6481 = property on="メイン測定ボタン_連続 3" class="Bool (指定)"("DisabledEnum"=w8450) -> ()  [unwired: 2 in, 2 out]
            }
            frame 3 {
              n6482 = property on="メイン測定ボタン_単発 4" class="Bool (指定)"("DisabledEnum"=w8451) -> ()  [unwired: 2 in, 2 out]
